vi "Main_03B.vi"() -> ()   [LabVIEW 2023]
uses:
  Cluster Digit.ctl
  <vilib>/Utility/miscctls.llb/LVMapReplaceAction.ctl
panel:
  out "Answer":i32
  out "Part Numbers":i32[](array[numeric])
  out "Answer":u32
  in  "Puzzle":string="................................................965..583........389.................307.................512......................395.....387\n........................#....374...382....250...*..........737*....*896.395...........*....................$.........................#......\n..494.........532-...474......*.......#....*...................522......*..........%...........................%...+................269.....\n.....*..#................506..143........375......77.....155...........400.518...64....773...718..797........694....972.603.....*...........\n....479.795...............*..........800...........*.$.......264*636.......@..............&..*...*.......499...............*...5.20.........\n515...................512.484...*....*...=......390...427...................................644.804.........*...@......-..532............28.\n..........607...........&.....105...906...910.......@............979.969...........-..=.............462....414..101.361..........283$.......\n..........*...781................................925..............=...*..........434..899....368.......*..................33...........*....\n.......850.......=........559..249...................732.....430....132........................*.....................817-.=.........613.381.\n....................157....*...&....978..............$......-...................*626.-.......297.............750............................\n..........312...........606........*....136.............593.............638...........177.....................*....672.772....998.491=......\n....450......*..156...............760.....=.......227......%..794...157........................919.......&....607..*...*....................\n.......*...108...............968...................-..........*........*....80....669..........$..........854......6..572.....743....&......\n......759.......649.............*832.......351.........433...418...997........*.....*.......46....187...........................*.....759...\n............344.&..........&.........573......@...556.............*..........884...748..317../....+..........................236............\n......#..................627.....334*..............*...933........774.534................*.......................................905........\n...642.....105..........................100.......372.....$...........*..........*982..527....$837..406.948....*127......455........*.......\n...........*.......383............293......*750.&.....774....630......51......826...........................361.........=.......993..822....\n....*..576.346.876....@..907.953..@..............982..*.........+.................913*782...*115..565..526........779.......971.............\n..20...*..........*.......*....%.............46-.......8................232................5.....................*....@........$........903.\n.....$.............483.....420......115....$......287...............................873.......................131....818...............*....\n......161....*362.....................-.266.........*......524...157.79....@.396.......*............848@.293............................988.\n..........412...................................97..721.....#.......*...638../......305.......................+.................630*818.....\n.194..................556....297.253...........*.........................................................@.....186..213..819................\n................154.....$.......*....454......46.795.686.......=..204.........$...=............771.....171..........#................-456...\n..................*.....................*........*.....-.....457.....*....638.466..579......................#..........109.....727..........\n..................177......785.769...827..........500....168........479....*...........=....255..............74...........*845....*..375....\n................-.........*.....*..........................*..............360..681......700.......................853...........781.....*...\n..846..91......966........511.435.............245.......617.............*.....*....................................$.....810...........836..\n.....*.................................%86......*..............121.......721..751......386*.......476*60...%195......801...%.......345......\n..763........+....428@....-40.391...............970......803......=...*....................351...................185....*.....118...*.......\n......#862..345....................629......45............+.........897.....802........488..........................*.....274.../..676../...\n..945.............299.......$......*..........................183..................190...&........763.....484..364...235....%..........564..\n...*..............*........404...527....&....137.814.......57......890.......407..*.........................*...*..............711&.........\n....424..........66..................966.......*.@.........*......*......806...+........................98....762......$...663........605...\n....................404......................614...489..........150....-..*........367...................*.........909.863...#........*.....\n.............%759...*...+....916.498...&.............*.551..........191..606...............797........391.......................=568...898..\n........2*........632.987......*....*.155.$2......412........................730...401.....#....438..........412*199........................\n..........729...............89.753...........364.........687....................*.....*86........*.............................%.....657....\n...............182./687.214.*.......................141..*....................$..620.......706%.368.....*.............758....694.971....*774\n.....617........*.........*..335....89....583.........*..378...945.....272...97......................264.817.............*........*..+......\n.../....*506.779...31..168..................*......732............*.../.....................957......................104.156...160..219.$...\n....789.............*....../........671...45....................982.&.......%.......$.......*...264.............386..*..................588.\n..................575.......192...../..................51*952.......264....655..=17..113...998.............932.......638..........24*.......\n...........@............@.......................................#................................650..........*734...........652.....278....\n........903.....=....805......944..............................377........477........&73.610.......+...640..........852.........*893........\n.............882.........@768..%..103........465......636.............................................*..........29...*.661.295......61.....\n.....................467.........$......292...*.........&..........640.......926.........201..173...38...........*..805.*.............*.....\n......296....317.......*.....995............$.889..890....665.......*....47..@....701&..$.......$......739....388.......257............790..\n..989..*.....&....980..168.....*...........17........*.....*.......894..*.........................*200.*....................................\n..../...561....................198.34*811......726.122...+.63..437......787.........668........355.......641....@...........................\n.................................................*.....112.....*................798*.......420..........*........244..758..............771..\n...&.......573..............515..................252........511......................396...%.......805.736............/..........546........\n342.......*....................*.44.................................*....399.188.....*........................254........13*................\n........%..720.............695......875*362.........@...649*919..585.477...*..*...245....450....-............*.......743....645.&......796..\n.....556.........460.........$..............919&....679...................935.............*...273.........396.........*..........659........\n...&.............-.........%.....542*...............................................255.368........387..............435..612*...............\n980................484...964.........736........%327.......210..+......962.610...............396.............492.............259.970*.......\n....-.......850...............645...........56.........275*.....928.....*.....-..81....133........=..889....*........................382....\n..382................419*.......*......@......*.............439........953.......*....*..........341..*..322.....226.342.......*598.........\n...............636=......662.204........620..13..............*...171..............19..396............27.............*.......539........278..\n.........131.........133........................282...900...48...*........678.379................+.....................798.......131....@...\n.....684*.....944.......*...@.....991...................*.........90.......*..+...818.783....19..492...501*842..........*..480*..@..........\n..........515..........855...646.+.......451.../533.....115...../.........841.................#........................272...........154....\n....107=..*................................&..........=.......631.....837.............52..............485......193.%.......983......*.......\n..........587............405*329....957............451............60.*............370......................222..*...461....@.......894..534.\n..705...............131...............$...640...............127*8.+..859.145.......%...440...%..................875.........................\n...*..714....783..........@986......&........*.........................................*...199.451....=.....................87.......190....\n.349..*......%.....429...............602..562..519................=......112*....669....8..............105...........#......../..387........\n.....792.............*.......854..............*.................93...........808...$...........%673........802$.......586..........*........\n.............-.......282.....+...-756.......291.........&...............................209.......................534.......573.831....*955.\n..........195............401..........617.............676.........................................961..716...................*..............\n.....762................*.......*864.........%694..............249./....-....572.327..........784..*..........@.534........883.........724..\n......%..............#...109.304....................................56...240.*...*......657...%....837..792.292...=...............*.........\n...................974..............89..............629....#460..............330.....*....*..............*................620#...887........\n...877*793..................680+...*........$662...*..............................365.898..773.........726...........607.............579....\n.................................316.404...........716.....*775.....%.........................................573.67.#...399.953......*.....\n.......931...................91@.....*.........680.....395.......760......165....302............960....*.........*.......*.........697......\n.......*......962..997/.............363.....*....*....@....126........566*........$..4..739*..........545.953.............955...............\n....548.........%................./.....*.734.....653.....*...........................#.....489..............*....336.763...................\n........@.185........88.........483...208......-..........419..331......460.../46.406.......................582.-....*..........408.........\n.....106../......654..*.....................423.......109.........*................*............269..%21.........632.....324+......*...*....\n................%....265......906....926.............*............475..60........188...............*.............................994..905...\n........=781....................*....*.....938....401.......857.......*.......................802.300..625.....207..%.......................\n..................355..894...410....402...*...................*.....467................660*..*.........%.......*....721.....&....764........\n...........554...*.......*..............277..-.......648.......491..........................968...........24....380......520....*...........\n......%....*.....757......788.................851......*...416.....493........635....241.........409.....*..........362......660............\n.......23..52..........@............................791.....*......+...=..*.........../...$209...*......282..214...=....370.................\n...................328..291.529.........................50.63........412.591..../..............169........................+........+........\n..701&....=..198.....*.........*....+...........896......$..../................772......*626........458..578=...............337..95...482...\n.......540...&......989....227..736.229.....................52...........241..........95.............*..................599...*......*......\n........................................820.397................937...664*...............................820...222.185...*.....47....862..192\n...........................$.....484.....*..$.......$601........*...............540.........&.............*..............694................\n.....818.630..........15..495...........119...36.........273.....329..=.398....*...........578....220...607..580.......%.......876..........\n.....*........=......*...................................*...........30..=......89..........................*.......182....574.$............\n...98...127....182.363..921..............................273.........................................@231..926...............=....=18.......\n........&.................................183........7@.......................347=.....=......903....................*732..............782..\n.............*635............................%.604*.........@.#910.226...............288..........767.............227............753/..*....\n770.......661............812...$709..430...........997....556......*.....................@...970...........949..........................775.\n............................................984.....................845.......$........861.......297..415.*...............789..*937.........\n..541.......614..10.........453.....................67.....................735...../..............*..*.......................*..............\n...%.../....*..........468...=........*824.109........*58............318............29.....152..538.488.....423.......19......602...162.....\n......279.363.228........*.........221.............&.......*..................................@................*788....*...........*........\n706....................114..............&987.873..316...701.871.....846...501......200.603..........876.................929......178........\n...*..503.......78.................................................-......*..........*............+.........179......$......................\n.850.....$..118...+.............944..........19.............@735..........388..160...365..582....524..........*.......355.....840...........\n..............*......*..........=...475+.926*.....433.............../146.......*..............................380.....................614...\n...........228....200.695..........................*..391..529..................918...290...340..16*.....482................363.........$...\n.......906......................993......=986...874...*...#....+............37...........*....=...........#...................*.....32......\n...&......*230..204=........721...*.$...............839.....456..553..601..*...408.....914..................77.................662..*..=554.\n...29.......................*...717.248.....358.................@......$...977...*................94.....................*846...............\n.............542..546.....52.................*........286........................669......................=...401......61.....709*389.480...\n........989......*....253....713.........742..171.........325....976....*...513/....................967.246....*........................*...\n...........=....571...*........-..=456.....................*........*..300.......344..........146..............87........................66.\n..199*................204..............+.490.......584...427.166...810.....431......+...115....*..........195...........=...................\n......247.645....................693.204....-.....*....................310...*..*........*.....772....686*.........=323.194....451......=...\n.....................596.304*696.@....................................*....220...351..444..934..................................+........136\n..736...............&..................................510..250..638.766..................*....511....195.........#..778..&902....721.......\n...........758............*..........=401......210..#.....&.-...*................572...385....*.......%.....200.248.*..............*........\n...........*...........991.358.256.........782*......742.........832....*.......=..........799...675*......*.........80.819.902...18........\n...........735...*.............*........*.......*242.....414*704.....194..325...........................569..............$...@..............\n..................772.......309...+..204.....659.....&.....................*............297*..396*494.......26......................131.....\n.....%..+.......................169...................860..333...212*....459.............................../.......392.............@.....103\n....628..891....../....519..88............................*..........530......90*....225.418....112....614....274..$......169%.399...481....\n850............829..48..%.........931........./388.......270..............@......798......#........@....*........$...............-..*.......\n...*876...............*...820.....*............................614*834...745............................575..................-......827.....\n......................764....*..432...........516$.133..633..................489$........396.255.............636..413*.811....337.......*682\n.667......................639...........199..........*...+......=....*500.........401@......*...........878-..*........../...........419....\n....@......28...........................*...#....@..72.......539..708........237.................=............675.851@......................\n.......777........406...459$..........993.445.719......./......................+...706........386....%....../..................*96.271......\n.311..*.......................&......................317../542....................@.....+.........136......821.543..........947.............\n...*..982.....657..70=..948#..159..777../.....757....................816...............887.............325........*....................871..\n.804..........=.....................*..284..........255*...............+....48...589*......199................#.68..542......&.&241...*.....\n.......10............604.....287...66......507..........917...585............-.......6.327..-......822.....718.....*.......825.......34.....\n........*......904$....*..................+......*.............*.....454.820............@.....492.*................887............@.........\n.......645.-.........49..............844.........533........958.........*.......32.892..........%.118...+..670*296......%...122..840.230....\n....=......176..........................*.=..........................%1.....397*...........820.........407...............21...........*.....\n...913...........&............408.....135.300..............775...993.........................@..............%.....272...........*626...101..\n..................95..505......*.................581.........+...*...........59*23.......449.......964...657.......*..........75............\n.............................87...622..........................822...............................................215.............810........"
  in  "Example":string="467..114..\n...*......\n..35..633.\n......#...\n617*......\n.....+.58.\n..592.....\n......755.\n...$.*....\n.664.598.."
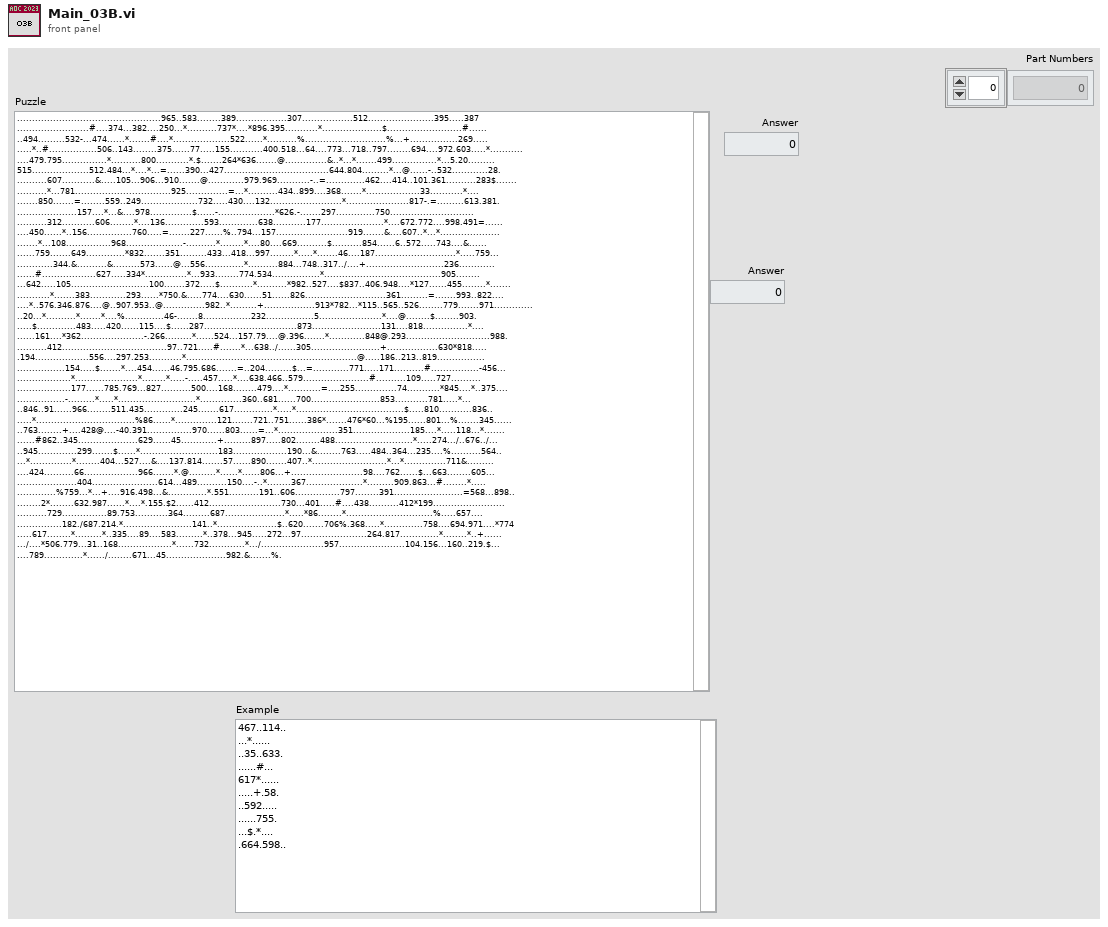
[diagram p1: front panel]
types:
  T1 = typedef "Cluster Digit.ctl" = cluster{"ascii":u8, "Row":i32, "Col":i32, "Digit":i32}
  T2 = typedef "LVMapReplaceAction.ctl" = enum32{"Modify Entry only if found", "Add or Modify Entry", "Delete Entry"}
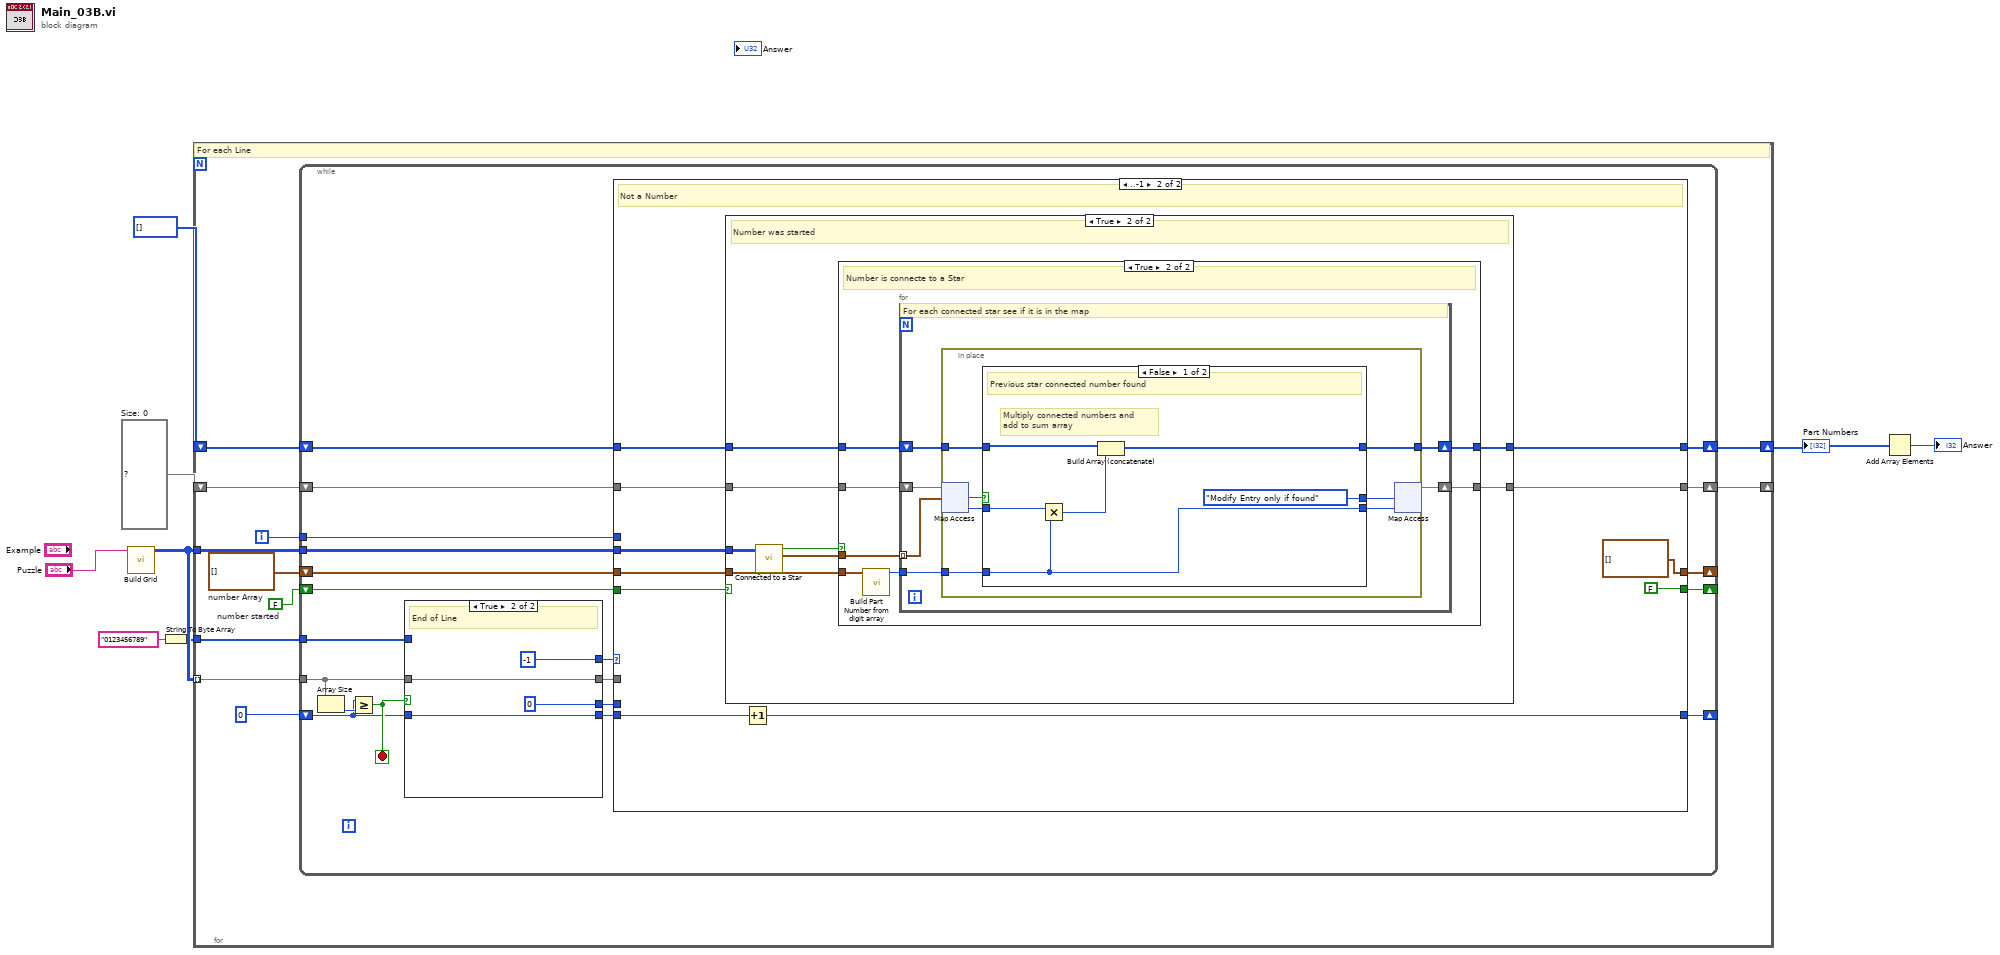
[diagram p0: block diagram]
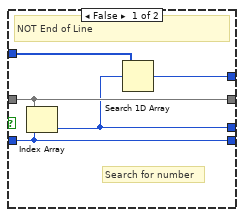
[diagram p2: hidden frame]
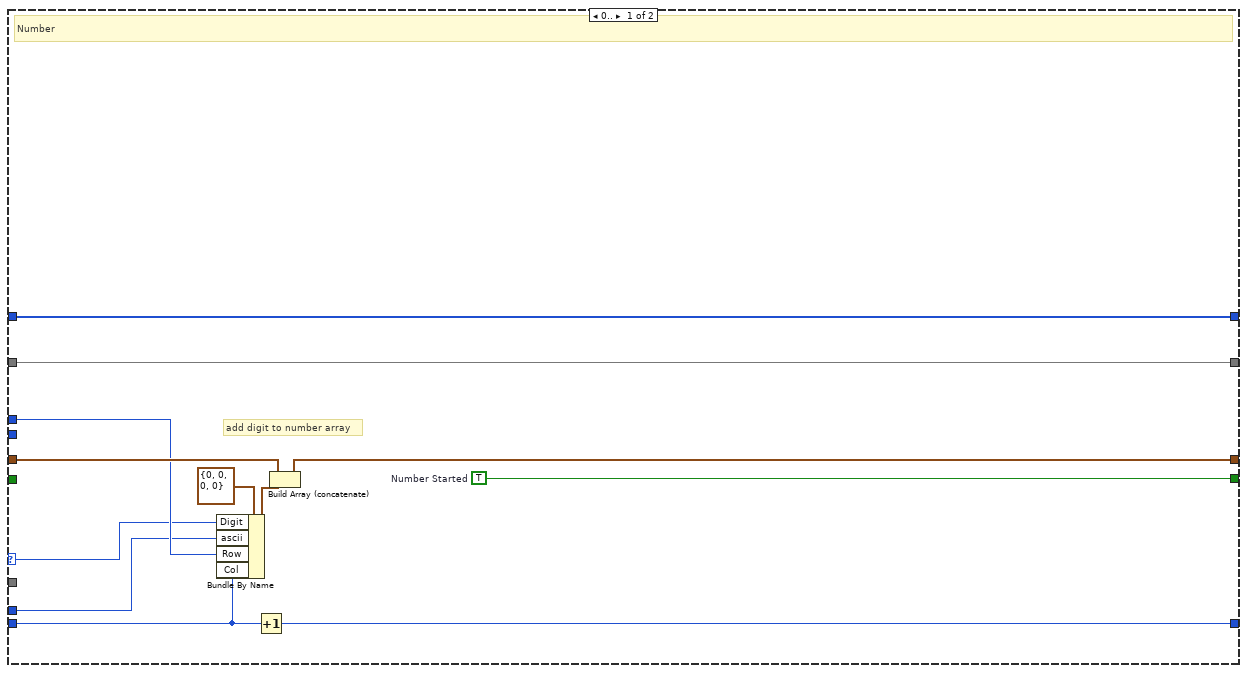
[diagram p3: hidden frame]
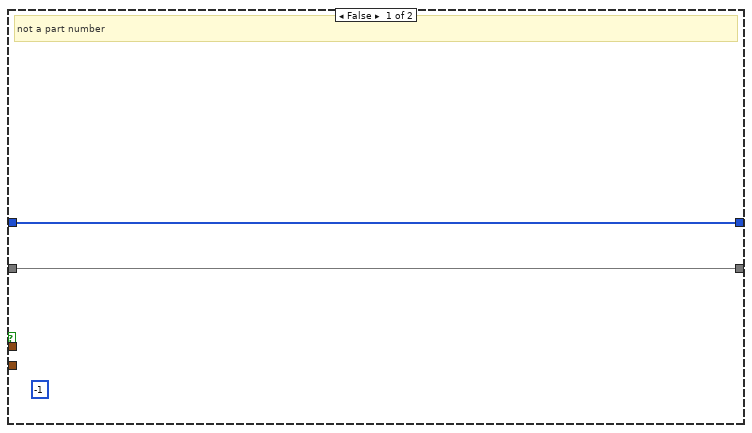
[diagram p5: hidden frame]
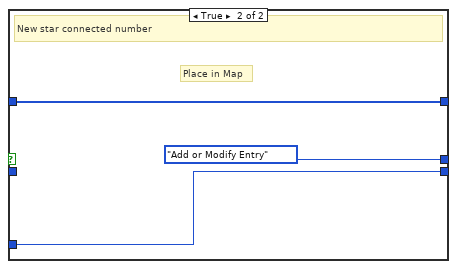
[diagram p6: hidden frame]
diagram:
  w4 = map{T1, i32} {}  # Size: 0
  n1 = call "Build Grid.vi"("string Grid"="Puzzle") -> ("unsigned byte array"=w8:u8[][])  [unwired: 10 in]
  n2 = String To Byte Array(string="0123456789" ("String")) -> (unsigned byte array=w6:u8[])
  n3 = for {
    tunnel: w8 -> [w19]
    tunnel: w8 -> [w18] mode=indexing
    tunnel: w6 -> [w13]
    shift-right: [w12] -> _
    shift-left: w4 -> [w11]
    shift-right: [w9] -> w2
    shift-left: i32[] [] ("Part Numbers") -> [w10]
    i -> [w15]
    w14 = T1[] []  # number Array
    w16 = FALSE  # number started
    # "For each Line"
    n4 = while {
      tunnel: w19 -> [w30]
      tunnel: w18 -> [w35]
      shift-right: [w36] -> _
      shift-left: 0 -> [w24]
      shift-right: [w28] -> _
      shift-left: w14 -> [w31]
      shift-right: [w37] -> _
      shift-left: w16 -> [w38]
      tunnel: w15 -> [w29]
      tunnel: w13 -> [w27]
      shift-right: [w22] -> w12
      shift-left: w11 -> [w23]
      shift-right: [w20] -> w9
      shift-left: w10 -> [w21]
      stop <- w34 stop-if-true
      n5 = Array Size(array=w35) -> (size(s)=w25:i32)
      n6 = Greater Or Equal?(x=w24, y=w25) -> (x >= y?=w34:bool)
      n7 = case shown="True" w34 {
        tunnel: [w44 -1 ("index of element")] -> w39
        tunnel: w35 -> [w42 w47]
        tunnel: w24 -> [w43 w48]
        tunnel: [w43 w48] -> w33
        tunnel: [w42 w47] -> w32
        tunnel: w27 -> [w40 _]
        tunnel: [w41 u8 0] -> w26
        frame False {
          # "Search for number"
          # "NOT End of Line"
          n8 = Index Array(array=w42, index=w43) -> (element=w41:u8)
          n9 = Search 1D Array(1D array=w40, element=w41) -> (index of element=w44:i32)  [unwired: 1 in]
        }
        frame True {
          # "End of Line"
        }
      }
      n10 = case shown="..-1" w39 {
        selector: w39 -> [w51 _]
        tunnel: w33 -> [w54 w71]
        tunnel: w38 -> [_ w69]
        tunnel: [w60 FALSE] -> w37
        tunnel: [w53 w70] -> w36
        tunnel: w32 -> [_ _]
        tunnel: w31 -> [w58 w68]
        tunnel: w30 -> [_ w67]
        tunnel: w29 -> [w55 _]
        tunnel: [w57 T1[] [] ("Digit")] -> w28
        tunnel: w26 -> [w52 _]
        tunnel: w23 -> [w50 w64]
        tunnel: [w50 w63] -> w22
        tunnel: w21 -> [w49 w62]
        tunnel: [w49 w61] -> w20
        frame 0.. {
          w60 = TRUE  # Number Started
          # "add digit to number array"
          # "Number"
          n11 = Bundle By Name(cluster=T1 {"ascii"=0, "Row"=0, "Col"=0, "Digit"=0} ("Digit"), "Digit"=w51, "ascii"=w52, "Row"=w55, "Col"=w54) -> (w56:T1)
          n12 = Increment(x=w54) -> (x+1=w53:i32)
          n13 = Build Array (concatenate)(w58, w56) -> (w57:T1[])
        }
        frame ..-1 {
          # "Not a Number"
          n14 = case shown="True" w69 {
            tunnel: w68 -> [_ w80]
            tunnel: w67 -> [_ w81]
            tunnel: w64 -> [w73 w78]
            tunnel: [w73 w77] -> w63
            tunnel: w62 -> [w72 w75]
            tunnel: [w72 w74] -> w61
            frame False {
              # "No Previous number"
            }
            frame True {
              # "Number was started"
              n15 = call "Connected to a Star.vi"("Digit Array"=w80, "Unsigned Byte Array"=w81) -> ("Connected Star Array"=w76:T1[], "Connected to Star"=w79:bool)  [unwired: 8 in]
              n16 = case shown="True" w79 {
                tunnel: w80 -> [_ w90]
                tunnel: w78 -> [w83 w88]
                tunnel: [w83 w87] -> w77
                tunnel: w76 -> [_ w86]
                tunnel: w75 -> [w82 w85]
                tunnel: [w82 w84] -> w74
                frame False {
                  (unwired) -1 ("Part Number Out")
                  # "not a part number"
                }
                frame True {
                  # "Number is connecte to a Star"
                  n17 = call "Build Part Number from digit array.vi"("Digit Array"=w90) -> ("Part Number Out"=w89:i32)  [unwired: 10 in]
                  n18 = for {
                    tunnel: w89 -> [w93]
                    shift-right: [w95] -> w87
                    shift-left: w88 -> [w96]
                    tunnel: w86 -> [w94] mode=indexing
                    shift-right: [w91] -> w84
                    shift-left: w85 -> [w92]
                    # "For each connected star see if it is in the map"
                    n19 = in-place {
                      in-place-border: w93 -> [w100]
                      in-place-border: w92 -> [w101]
                      in-place-border: [w97] -> w91
                      n20 = in-place-map #1(w96, w94) -> (w99:i32, w102:bool)  [unwired: 1 in]
                      n21 = case shown="False" w102 {
                        tunnel: [LVMapReplaceAction."Modify Entry only if found" ("action") LVMapReplaceAction."Add or Modify Entry" ("action")] -> w103
                        tunnel: w101 -> [w106 w110]
                        tunnel: w100 -> [w107 w111]
                        tunnel: w99 -> [w108 _]
                        tunnel: [w107 w111] -> w98
                        tunnel: [w104 w110] -> w97
                        frame False {
                          # "Multiply connected numbers and\nadd to sum array"
                          # "Previous star connected number found"
                          n22 = Multiply(x=w108, y=w107) -> (x*y=w105:i32)
                          n23 = Build Array (concatenate)(w106, w105) -> (w104:i32[])
                        }
                        frame True {
                          # "Place in Map"
                          # "New star connected number"
                        }
                      }
                      n24 = in-place-map #1(w98, w103) -> (w95:map{T1, i32})  [unwired: 2 out]
                    }
                  }
                }
              }
            }
          }
          n25 = Increment(x=w71) -> (x+1=w70:i32)
        }
      }
    }
  }
  "Part Numbers" <- w2
  n26 = Add Array Elements(numeric array=w2) -> (sum=→"Answer":i32)
